vi "daqio_Get_All_Events.vi"(8 "error in (no error)":errorcluster, 11 "daq.io type in":T2={"daq.io ref"=refnum, "daq.io API Base"="http://dashboard.daq.io/api/v1", "Device Type Key"="", "Device Key"="", "Account ID"=""}) -> (0 "error out":errorcluster, 1 "Events":T1[](array[typedef]), 3 "daq.io type out":T2={"daq.io ref"=refnum, "daq.io API Base"="http://dashboard.daq.io/api/v1", "Device Type Key"="", "Device Key"="", "Account ID"=""})   [LabVIEW 2013, in "daqio minimal.lvlib"]
doc: "This VI returns all Tags for a specific device."
uses:
  daqio minimal.lvlib
  _typedefs/daqio-Type.ctl
  <vilib>/httpClient/ClientHandle.ctl
  _typedefs/daqio-Event-Def.ctl
  <vilib>/Easy HTTP Client/Easy HTTP.lvlib
  <vilib>/httpClient/LabVIEWHTTPClient.lvlib
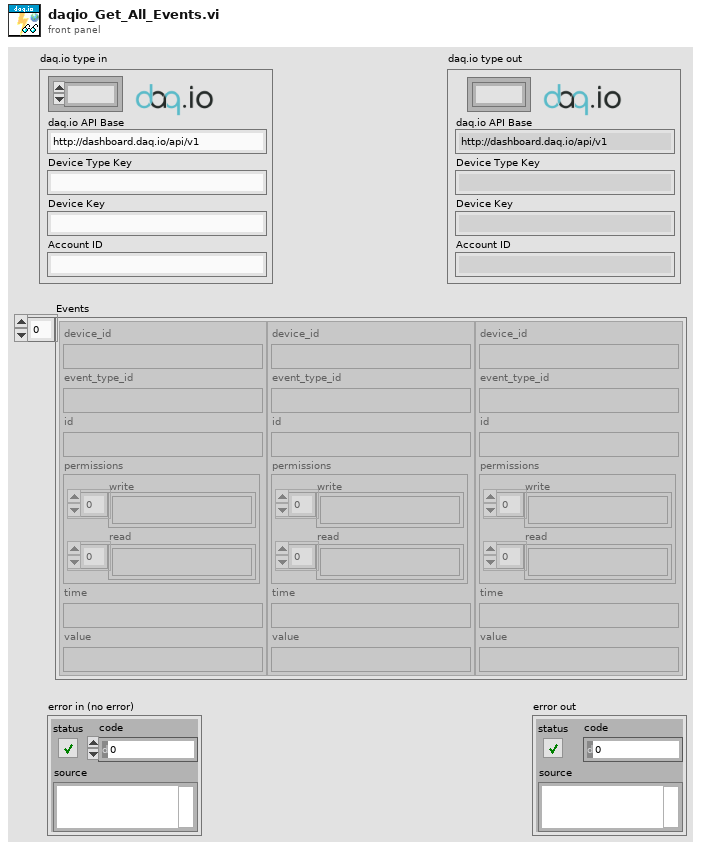
[diagram p1: front panel]
types:
  T1 = typedef "daqio minimal.lvlib/daqio-Event-Def.ctl" = cluster{"device_id":string, "event_type_id":string, "id":string, "permissions":cluster{"write":string[], "read":string[]}, "time":string, "value":string}
  T2 = typedef "daqio minimal.lvlib/daqio-Type.ctl" = cluster{"daq.io ref":T3, "daq.io API Base":string, "Device Type Key":string, "Device Key":string, "Account ID":string}
  T3 = typedef "LabVIEWHTTPClient.lvlib/ClientHandle.ctl" = refnum<k1>
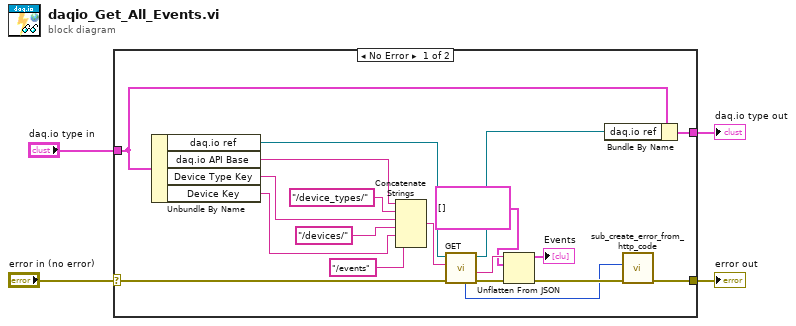
[diagram p0: block diagram]
diagram:
  n1 = case shown="No Error" "error in (no error)" {
    selector: "error in (no error)" -> [w15 w24]
    tunnel: "daq.io type in" -> [w21 w25]
    tunnel: [w20 w25] -> w3
    tunnel: [w18 w24] -> w2
    frame No Error {
      n2 = Unbundle By Name(w21) -> ("daq.io ref"=w17:T3, "daq.io API Base"=w19:string, "Device Type Key"=w10:string, "Device Key"=w9:string)
      n3 = Concatenate Strings(w19, "/device_types/", w10, "/devices/", w9, "/events" ("string")) -> (w8:string)
      n4 = call <vilib>:"GET.vi"("error in (no error)"=w15, "url"=w8, "client handle"=w17) -> ("error out"=w13:errorcluster, "body"=w14:string, "client handle out"=w16:T3, "HTTP Response Code"=w11:i32)  [unwired: 4 in, 1 out]
      n5 = Unflatten From JSON(JSON string=w14, type and defaults=T1[] [], error in (no error)=w13) -> (value=→"Events":T1[], error out=w12:errorcluster)  [unwired: 4 in]
      n6 = Bundle By Name(cluster=w21, "daq.io ref"=w16) -> (w20:T2)
      n7 = call "sub_create_error_from_http_code.vi"("error in (no error)"=w12, "HTTP Code"=w11) -> ("error out"=w18:errorcluster)  [unwired: 8 in, 1 out]
    }
    frame Error {
    }
  }
  "error out" <- w2
  "daq.io type out" <- w3
